vi "GdsLanguage_RemoveNullCharsInString.vi"(2 "StringArray-IN":string[](array[string]), 3 "MaxLengthLimit(ignored if not wired)":i32, 4 "MinLengthLimit(ignored if not wired)":i32) -> (16 "StringArray-Out":string[](array[string]))   [LabVIEW 2020]
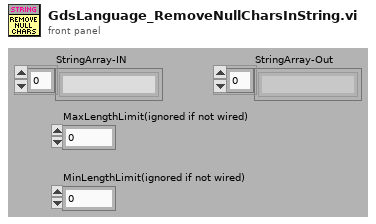
[diagram p1: front panel]
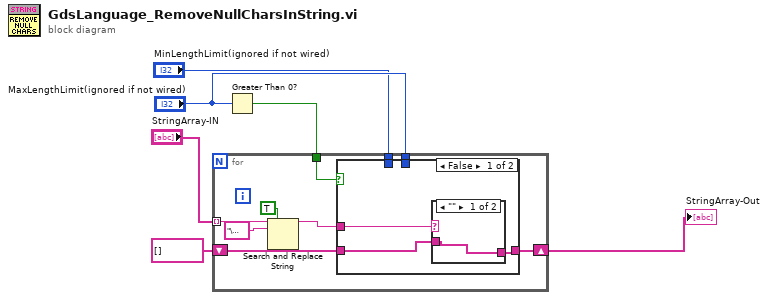
[diagram p0: block diagram]
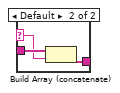
[diagram p2: hidden frame]
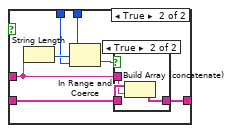
[diagram p3: hidden frame]
diagram:
  n1 = Greater Than 0?(x="MaxLengthLimit(ignored if not wired)") -> (x > 0?=w3:bool)
  n2 = for {
    tunnel: "StringArray-IN" -> [w15] mode=indexing
    shift-right: [w12] -> w6
    shift-left: string[] [] -> [w11]
    tunnel: w3 -> [w9]
    tunnel: "MaxLengthLimit(ignored if not wired)" -> [w8]
    tunnel: "MinLengthLimit(ignored if not wired)" -> [w7]
    n3 = Search and Replace String(replace all?=TRUE ("replace all? (F)"), input string=w15, search string="\u0000") -> (result string=w10:string)  [unwired: 5 in, 3 out]
    n4 = case shown="False" w9 {
      tunnel: [w17 w29] -> w12
      tunnel: w11 -> [w18 w28]
      tunnel: w10 -> [w16 w27]
      tunnel: w8 -> [_ w24]
      tunnel: w7 -> [_ w25]
      frame False {
        n5 = case shown="\"\"" w16 {
          selector: w16 -> [_ w20]
          tunnel: w18 -> [w19 w22]
          tunnel: [w19 w21] -> w17
          frame "" {
          }
          frame Default {
            n6 = Build Array (concatenate)(w22, w20) -> (w21:string[])
          }
        }
      }
      frame True {
        n7 = String Length(string=w27) -> (length=w26:i32)
        n8 = In Range and Coerce(upper limit=w24, x=w26, lower limit=w25) -> (In Range?=w23:bool)  [unwired: 1 out]
        n9 = case shown="True" w23 {
          tunnel: [w30 w32] -> w29
          tunnel: w28 -> [w30 w33]
          tunnel: w27 -> [_ w31]
          frame False {
          }
          frame True {
            n10 = Build Array (concatenate)(w33, w31) -> (w32:string[])
          }
        }
      }
    }
  }
  "StringArray-Out" <- w6
